vi "20TVTI-Set-Htr-Dewar.vi"(8 "error in (no error)":errorcluster, 10 "VTI Control":T1={"Set VTI SP"=TRUE, "Change NV Status"=TRUE, "Set NV Setpoint"=TRUE, "Change Heater Status"=FALSE, "Set D-Heater Setpoint"=FALSE, "Set Heater Setpoint"=FALSE, "Change D-Heater Status"=FALSE, "Set Sweep Type"=FALSE, "Setpoint (K)"=0.0, "Rate (K/min)"=0.0, "Setpoint Heater"=0.0, "Setpoint D-Heater"=0.0, "Setpoint NV"=0.0}, 11 "Mercury Reference In":T2) -> (0 "error out":errorcluster)   [LabVIEW 2016]
uses:
  Equipment/Mercury iXX/Public/Controls/Mercury Reference.ctl
  Equipment/Mercury iXX/Public/Controls/Comms Transport Layer.ctl
  Equipment/Mercury iXX/Private/Controls/Query Dynamic Reference.ctl
  Gustav/20TVTI_Control.ctl
  Equipment/Mercury iXX/Public/Libraries/Pressure/Open/Open Pressure Device.vi
  Equipment/Mercury iXX/Mercury iXX.lvlib
  Equipment/Mercury iXX/Public/Libraries/Pressure.lvlib
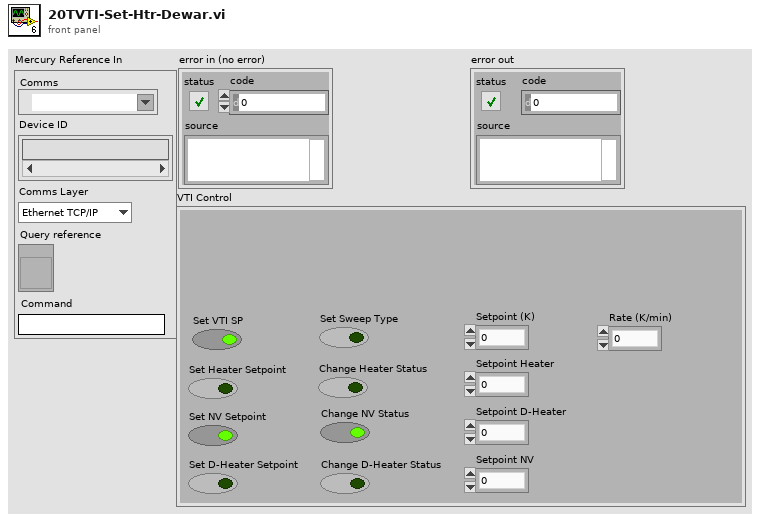
[diagram p1: front panel]
types:
  T1 = typedef "20TVTI_Control.ctl" = cluster{"Set VTI SP":bool, "Change NV Status":bool, "Set NV Setpoint":bool, "Change Heater Status":bool, "Set D-Heater Setpoint":bool, "Set Heater Setpoint":bool, "Change D-Heater Status":bool, "Set Sweep Type":bool, "Setpoint (K)":dbl, "Rate (K/min)":dbl, "Setpoint Heater":dbl, "Setpoint D-Heater":dbl, "Setpoint NV":dbl}
  T2 = typedef "Mercury iXX.lvlib/Mercury Reference.ctl" = cluster{"Comms":refnum<visa-resource-name>, "Device ID":string[], "Comms Layer":T3, "Command":string, "Query reference":T4}
  T3 = typedef "Mercury iXX.lvlib/Comms Transport Layer.ctl" = enum16{"Ethernet TCP/IP", "USB", "ISOBus - RS-232", "GPIB"}
  T4 = typedef "Mercury iXX.lvlib/Query Dynamic Reference.ctl" = refnum<vi>
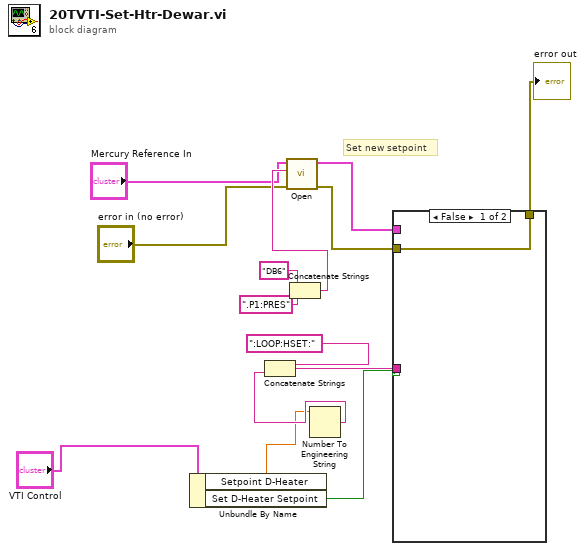
[diagram p0: block diagram]
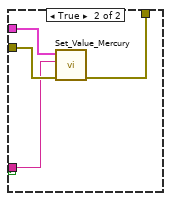
[diagram p2: hidden frame]
diagram:
  # "Set new setpoint"
  n1 = Unbundle By Name("VTI Control") -> ("Setpoint D-Heater"=w1:dbl, "Set D-Heater Setpoint"=w7:bool)
  n2 = Concatenate Strings("DB6", ".P1:PRES" ("Device Identifier")) -> (w9:string)
  n3 = call-poly "Open.vi"("error in (no error)"="error in (no error)", "Device Identifier"=w9, "Mercury Reference In"="Mercury Reference In") -> ("error out"=w13:errorcluster, "Mercury Reference Out"=w14:T2)  [unwired: 2 in, 5 out]
  n4 = Number To Engineering String(4:w1) -> (0:w2:string)  [unwired: 3 in]
  n5 = Concatenate Strings(":LOOP:HSET:", w2) -> (w8:string)
  n6 = case shown="False" w7 {
    tunnel: w14 -> [_ w19]
    tunnel: w13 -> [w15 w18]
    tunnel: [w15 w17] -> w4
    tunnel: w8 -> [_ w16]
    frame False {
    }
    frame True {
      n7 = call "Set_Value_Mercury.vi"("error in"=w18, "Noun(s)"=w16, "Mercury Reference In"=w19) -> ("error out"=w17:errorcluster)  [unwired: 7 in, 1 out]
    }
  }
  "error out" <- w4
